vi "Actual Flow SI.vi"(8 "Error In":errorcluster, 10 "Channel (0)":i32, 11 "VISA resource name":refnum<visa-resource-name>) -> (0 "Error Out":errorcluster, 1 "Flow":dbl[unit], 3 "dup VISA resource name":refnum<visa-resource-name>)   [LabVIEW 2016, in "MGC647C.lvlib"]
doc: "Return actual flow in SI unit.\n\n<b>Assuming:</b> Gas = N2. You need to take the gas correction factor into account ypurself!\n\n<b>Remember:</b> 1 ft^3/min = 28.32 l/min."
uses:
  MGC647C.lvlib
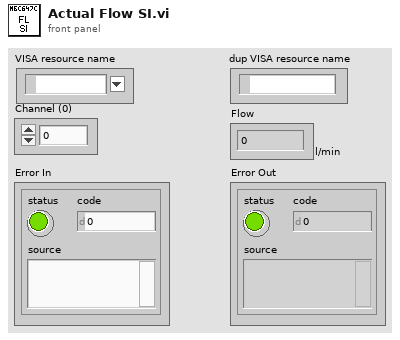
[diagram p1: front panel]
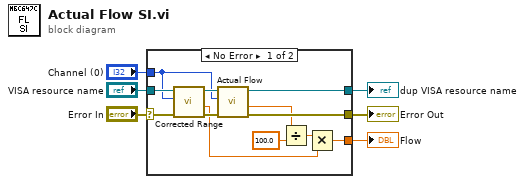
[diagram p0: block diagram]
diagram:
  n1 = case shown="No Error" "Error In" {
    selector: "Error In" -> [w12 w20]
    tunnel: "VISA resource name" -> [w10 w19]
    tunnel: [w14 w19] -> w5
    tunnel: [w15 w20] -> w4
    tunnel: [w16 _] -> w2
    tunnel: "Channel (0)" -> [w8 _]
    frame No Error {
      n2 = call "Corrected Range.vi"("Error In"=w12, "Channel (0)"=w8, "VISA resource name"=w10) -> ("Error Out"=w11:errorcluster, "Corrected Range"=w7:dbl[unit], "dup VISA resource name"=w9:refnum<visa-resource-name>)  [unwired: 6 in]
      n3 = call "Actual Flow.vi"("Error In"=w11, "Channel (0)"=w8, "VISA resource name"=w9) -> ("Error Out"=w15:errorcluster, "Actual Flow"=w13:dbl, "dup VISA resource name"=w14:refnum<visa-resource-name>)  [unwired: 6 in]
      n4 = Divide(x=w13, y=100.0) -> (x/y=w17:dbl)
      n5 = Multiply(x=w17, y=w7) -> (x*y=w16:dbl[unit])
    }
    frame Error {
    }
  }
  "dup VISA resource name" <- w5
  "Error Out" <- w4
  "Flow" <- w2
